vi "Read2ByteReg.vi"(7 "MxID":u8=254 format="%x", 8 "error in":errorcluster, 11 "RegAddr":u8=6 format="%x") -> (0 "error out":errorcluster, 3 "Data":u8[](array[numeric]) format="%x")   [LabVIEW 2014]
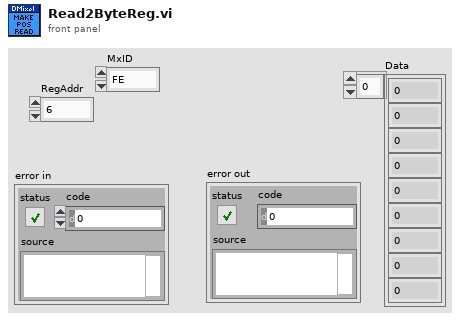
[diagram p1: front panel]
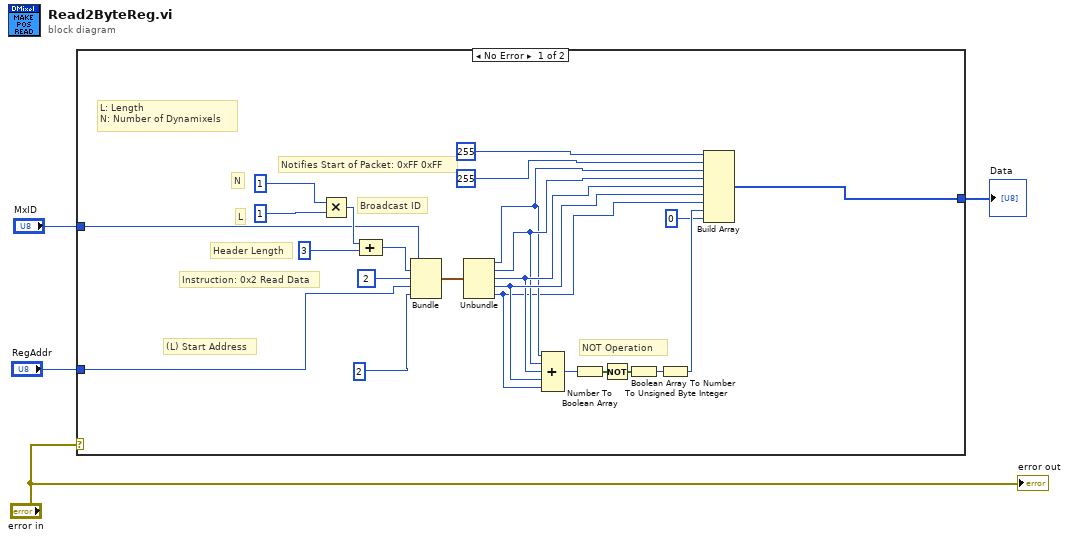
[diagram p0: block diagram]
diagram:
  n1 = case shown="No Error" "error in" {
    tunnel: "RegAddr" -> [w9 _]
    tunnel: [w15 _] -> w2
    tunnel: "MxID" -> [w10 _]
    frame No Error {
      # "L"
      # "NOT Operation"
      # "L: Length \nN: Number of Dynamixels"
      # "Header Length"
      # "N"
      # "(L) Start Address"
      # "Instruction: 0x2 Read Data"
      # "Broadcast ID"
      # "Notifies Start of Packet: 0xFF 0xFF"
      n2 = Multiply(x=u8 1 ("N"), y=u8 1) -> (x*y=w28:u8)
      n3 = Compound Arithmetic op=unknown(w28, u8 3 ("value")) -> (w27:u8)
      n4 = Bundle("MxID"=w10, w27, u8 2, "RegAddr"=w9, "x"=u8 2) -> (w23:cluster{"MxID":u8, u8, u8, "RegAddr":u8, "x":u8})  [unwired: 1 in]
      n5 = Unbundle(w23) -> ("MxID"=w11:u8, w12:u8, w13:u8, "RegAddr"=w14:u8, "x"=w7:u8)
      n6 = Compound Arithmetic op=ADD(w11, w12, w13, w14, w7) -> (w19:u8)
      n7 = Number To Boolean Array(number=w19) -> (Boolean array=w20:bool[])
      n8 = Not(x=w20) -> (.not. x?=w21:bool[])
      n9 = Boolean Array To Number(Boolean array=w21) -> (number=w22:u8)
      n10 = To Unsigned Byte Integer(number=w22) -> (unsigned 8bit integer=w6:u8)
      n11 = Build Array(u8 255, u8 255, w11, w12, w13, w14, w7, w6, u8 0 ("element")) -> (w15:u8[])
    }
    frame Error {
    }
  }
  "Data" <- w2
  "error out" <- "error in"
